vi "FilterRudder.vi"(10 "Notifier in":refnum<notifier>, 11 "Queue in 2":refnum<queue>) -> ()   [LabVIEW 2013]
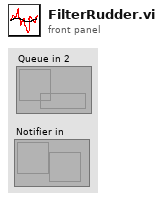
[diagram p1: front panel]
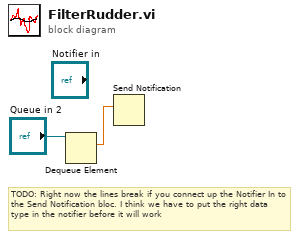
[diagram p0: block diagram]
diagram:
  # "TODO: Right now the lines break if you connect up the Notifier In to the Send Notification bloc. I think we have to put the right data type in the notifier before it will work"
  n1 = Dequeue Element(queue="Queue in 2") -> (element=w2:dbl)  [unwired: 2 in, 3 out]
  n2 = Send Notification(notification=w2) -> ()  [unwired: 2 in, 2 out]
